vi "LIA SOS Simulator.vi"() -> ()   [LabVIEW 2017]
uses:
  Cascaded-SOS/FPGA/Controls/IIR_Coeffs.ctl
  <instrlib>/_niInstr/DSP/v1/Shared/Public/IQ Data.ctl
  <vilib>/measure/maspectr.llb/FFT Power Spectrum and PSD for 1 Chan (CDB).vi
  <vilib>/Analysis/NI_AALBase.lvlib
  <vilib>/measure/NI_MAPro.lvlib
  <instrlib>/_niInstr/DSP/v1/Shared/niInstr DSP v1 Shared.lvlib
panel:
  out "size(s)":i32
  in  "Decimation (-1)":dbl=4.0 format="%#_p"
  out "Numeric":i32
  out "Waveform Graph 3":dbl[][](graph)
  out "Waveform Graph 2":cluster{"f0":dbl, "df":dbl, "magnitude":dbl[]}(graph)
  in  "IIR 2 coeffs":T1={"b0"=0.001556396484375, "b1"=-0.000762939453125, "-a1"=1.9305267333984375, "-a2"=-0.9328765869140625}
  out "Waveform Graph":cluster{"f0":dbl, "df":dbl, "magnitude":dbl[]}(graph)
  in  "Sampling Rate":dbl=1.0 format="%#_p"
  out "FFT Gain":dbl
  out "Noise (W|50ohms)":dbl
  out "k":dbl
  out "Noise vrms":dbl
  in  "Desired SNR (dB)":dbl format="%#_p"
  in  "Oscillator Magnitude":dbl=1.0 format="%#_13g"
  in  "Oscillator Frequency":dbl=0.001 format="%#_p"
  in  "Signal Offset":cdb format="%#_13g"
  in  "Singal Amplitude":dbl=0.5 format="%#_13g"
  in  "Signal Frequency":dbl=0.001 format="%#_p"
  in  "Number Samples":i32=10000
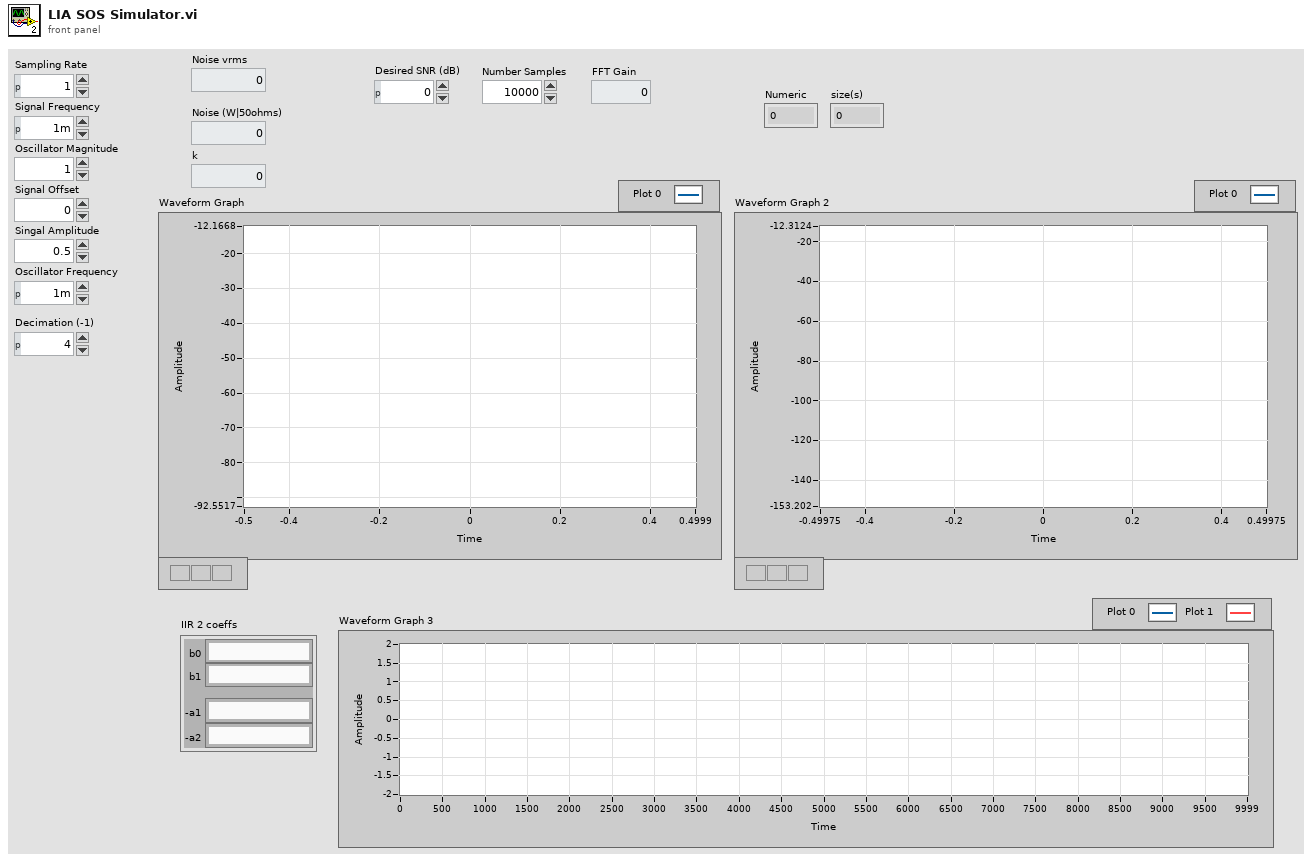
[diagram p1: front panel]
types:
  T1 = typedef "IIR_Coeffs.ctl" = cluster{"b0":fxp<+/-,18,2>, "b1":fxp<+/-,18,2>, "-a1":fxp<+/-,18,2>, "-a2":fxp<+/-,18,2>}
  T2 = typedef "niInstr DSP v1 Shared.lvlib/IQ Data.ctl" = cluster{"I":fxp<+/-,18,1>, "Q":fxp<+/-,18,1>, "overflow":bool}
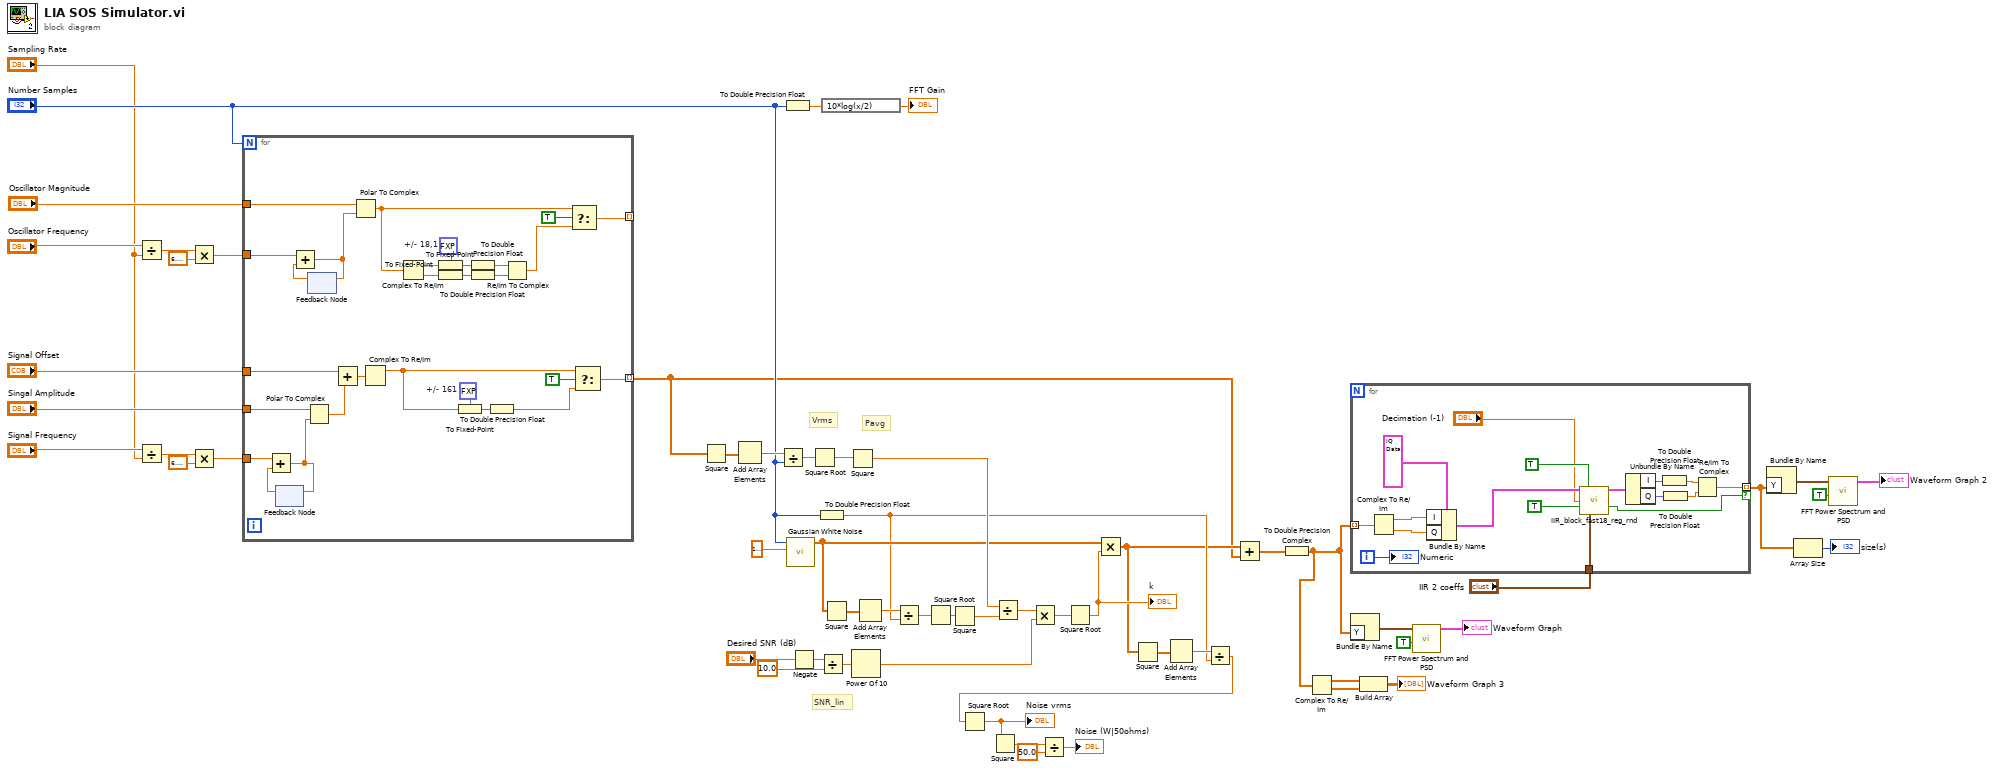
[diagram p0: block diagram]
diagram:
  # "SNR_lin"
  # "Pavg"
  # "Vrms"
  n1 = Divide(x="Oscillator Frequency", y="Sampling Rate") -> (x/y=w53:dbl)
  n2 = Divide(x="Signal Frequency", y="Sampling Rate") -> (x/y=w57:dbl)
  n3 = Multiply(x=w53, y=6.283185307179586) -> (x*y=w50:dbl)
  n4 = Multiply(x=w57, y=6.283185307179586) -> (x*y=w56:dbl)
  n5 = for {
    N: "Number Samples" -> [_]
    tunnel: w56 -> [w83]
    tunnel: "Singal Amplitude" -> [w86]
    tunnel: "Signal Offset" -> [w85]
    tunnel: [w69] -> _ mode=indexing
    tunnel: [w63] -> w15 mode=indexing
    tunnel: w50 -> [w74]
    tunnel: "Oscillator Magnitude" -> [w72]
    w64 = fxp<+/-,16,1> 0.0  # +/- 161
    w79 = fxp<+/-,18,1> 0.0  # +/- 18,1
    n6 = feedback #1() -> (w87:dbl)  [unwired: 1 in]
    n7 = Add(x=w83, y=w87) -> (x+y=w82:dbl)
    n8 = feedback-in #1(w82) -> ()
    n9 = Polar To Complex(1:w82, 2:w86) -> (0:w84:cdb)
    n10 = feedback #2() -> (w73:dbl)  [unwired: 1 in]
    n11 = Add(x=w74, y=w73) -> (x+y=w71:dbl)
    n12 = feedback-in #2(w71) -> ()
    n13 = Add(x=w85, y=w84) -> (x+y=w61:cdb)
    n14 = Polar To Complex(1:w71, 2:w72) -> (0:w70:cdb)
    n15 = Complex To Re/Im(x + iy=w61) -> (x=w60:dbl)  [unwired: 1 out]
    n16 = Complex To Re/Im(x + iy=w70) -> (x=w81:dbl, y=w80:dbl)
    n17 = To Fixed-Point(fixed-point type=w79, number=w81) -> (fixed-point=w78:fxp<+/-,18,1>)
    n18 = To Fixed-Point(fixed-point type=w79, number=w80) -> (fixed-point=w77:fxp<+/-,18,1>)
    n19 = To Fixed-Point(fixed-point type=w64, number=w60) -> (fixed-point=w65:fxp<+/-,16,1>)
    n20 = To Double Precision Float(number=w78) -> (double precision float=w76:dbl)
    n21 = To Double Precision Float(number=w77) -> (double precision float=w75:dbl)
    n22 = To Double Precision Float(number=w65) -> (double precision float=w62:dbl)
    n23 = Re/Im To Complex(1:w75, 2:w76) -> (0:w68:cdb)
    n24 = Select(t=w70, s=TRUE, f=w68) -> (s? t:f=w69:cdb)
    n25 = Select(t=w60, s=TRUE, f=w62) -> (s? t:f=w63:dbl)
  }
  n26 = Square(x=w15) -> (x^2=w48:dbl[])
  n27 = Add Array Elements(numeric array=w48) -> (sum=w47:dbl)
  n28 = Divide(x=w47, y="Number Samples") -> (x/y=w46:dbl)
  n29 = To Double Precision Float(number="Number Samples") -> (double precision float=w20:dbl)
  n30 = call <vilib>:"Gaussian White Noise.vi"("standard deviation"=1.0000000000000002, "samples"="Number Samples") -> ("Gaussian noise pattern"=w30:dbl[])  [unwired: 8 in, 1 out]
  n31 = Negate(x="Desired SNR (dB)") -> (-x=w33:dbl)
  n32 = Square Root(x=w46) -> (sqrt(x)=w45:dbl)
  n33 = To Double Precision Float(number="Number Samples") -> (double precision float=w18:dbl)
  n34 = Divide(x=w33, y=10.0) -> (x/y=w41:dbl)
  n35 = expression code="10*log(x/2)"(w20) -> (→"FFT Gain":dbl)
  n36 = Square(x=w30) -> (x^2=w37:dbl[])
  n37 = Square(x=w45) -> (x^2=w36:dbl)
  n38 = Power Of 10(x=w41) -> (10^x=w32:dbl)
  n39 = Add Array Elements(numeric array=w37) -> (sum=w38:dbl)
  n40 = Divide(x=w38, y=w18) -> (x/y=w39:dbl)
  n41 = Square Root(x=w39) -> (sqrt(x)=w40:dbl)
  n42 = Square(x=w40) -> (x^2=w35:dbl)
  n43 = Divide(x=w36, y=w35) -> (x/y=w34:dbl)
  n44 = Multiply(x=w34, y=w32) -> (x*y=w31:dbl)
  n45 = Square Root(x=w31) -> (sqrt(x)=w29:dbl)
  "k" <- w29
  n46 = Multiply(x=w30, y=w29) -> (x*y=w16:dbl[])
  n47 = Square(x=w16) -> (x^2=w28:dbl[])
  n48 = Add Array Elements(numeric array=w28) -> (sum=w27:dbl)
  n49 = Divide(x=w27, y=w18) -> (x/y=w26:dbl)
  n50 = Square Root(x=w26) -> (sqrt(x)=w25:dbl)
  "Noise vrms" <- w25
  n51 = Square(x=w25) -> (x^2=w24:dbl)
  n52 = Divide(x=w24, y=50.0) -> (x/y=→"Noise (W|50ohms)":dbl)
  n53 = Add(x=w16, y=w15) -> (x+y=w14:dbl[])
  n54 = To Double Precision Complex(1:w14) -> (0:w6:cdb[])
  n55 = Complex To Re/Im(x + iy=w6) -> (x=w5:dbl[], y=w4:dbl[])
  n56 = Bundle By Name("Y"=w6) -> (w13:waveform(cdb))  [unwired: 1 in]
  n57 = for {
    tunnel: w6 -> [w102] mode=indexing
    tunnel: [w94] -> w2 mode=indexing if=w93
    tunnel: "IIR 2 coeffs" -> [w92]
    i -> [w91]
    n58 = Complex To Re/Im(x + iy=w102) -> (x=w101:dbl, y=w100:dbl)
    n59 = Bundle By Name(cluster=T2 {"I"=0.0, "Q"=0.0, "overflow"=FALSE} ("IQ_Data_In"), "I"=w101, "Q"=w100) -> (w90:T2)
    n60 = call "IIR_block_fast18_reg_rnd.vi"("IQ_Data_In"=w90, "enable"=TRUE, "Decimation Factor (-1)"="Decimation (-1)", "Valid In"=TRUE, "IIR 2 coeffs"=w92) -> ("IQ_Data_Out"=w89:T2, "output valid"=w93:bool)  [unwired: 9 in]
    n61 = Unbundle By Name(w89) -> ("I"=w98:fxp<+/-,18,1>, "Q"=w97:fxp<+/-,18,1>)
    n62 = To Double Precision Float(number=w98) -> (double precision float=w96:dbl)
    n63 = To Double Precision Float(number=w97) -> (double precision float=w95:dbl)
    n64 = Re/Im To Complex(1:w95, 2:w96) -> (0:w94:cdb)
    "Numeric" <- w91
  }
  n65 = Build Array(w5, w4) -> (→"Waveform Graph 3":dbl[][])
  n66 = call-poly <vilib>:"FFT Power Spectrum and PSD.vi"("dB On (F)"=TRUE, "time signal"=w13) -> ("Power Spectrum / PSD"=→"Waveform Graph":cluster{"f0":dbl, "df":dbl, "magnitude":dbl[]})  [unwired: 6 in, 3 out]
  n67 = Bundle By Name("Y"=w2) -> (w8:waveform(cdb))  [unwired: 1 in]
  n68 = Array Size(array=w2) -> (size(s)=→"size(s)":i32)
  n69 = call-poly <vilib>:"FFT Power Spectrum and PSD.vi"("dB On (F)"=TRUE, "time signal"=w8) -> ("Power Spectrum / PSD"=→"Waveform Graph 2":cluster{"f0":dbl, "df":dbl, "magnitude":dbl[]})  [unwired: 6 in, 3 out]
